vi "Joint Manipulator Inertia.vi"   [LabVIEW 2017, in "NI_Kinematics.lvlib"]
doc: "Calculates a matrix that represents the kinetic energy of the end effector of a robotic arm in joint space. Wire data to the <B>joint positions</B> input to determine the polymorphic instance to use or manually select the instance. \n\n<B>.m file:</B> inertia"
uses:
  <vilib>/robotics/Kinematics/NI_Kinematics.lvlib
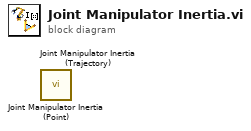
[diagram p0: block diagram]
diagram:
  n1 = call <vilib>:"Joint Manipulator Inertia (Point).vi"() -> ()  [unwired: 9 in, 3 out]
  n2 = call <vilib>:"Joint Manipulator Inertia (Trajectory).vi"() -> ()  [unwired: 9 in, 3 out]
